vi "SecToCost.vi"(10 "Rate":dbl, 11 "Seconds":dbl) -> (3 "StoCcluster":T1)   [LabVIEW 2024]
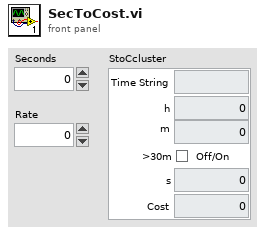
[diagram p1: front panel]
types:
  T1 = cluster{"Time String":string, "h":i32, "m":i32, ">30m":bool, "s":i32, "Cost":dbl}
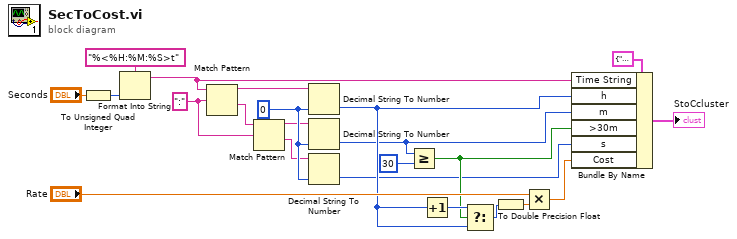
[diagram p0: block diagram]
diagram:
  w13 = ":" ("regular expression")
  w17 = 0 ("default (0 I32)")
  n1 = To Unsigned Quad Integer(1:"Seconds") -> (0:w10:u64)
  n2 = Format Into String(format string="%<%H:%M:%S>t", w10) -> (resulting string=w7:string)  [unwired: 2 in, 1 out]
  n3 = Match Pattern(string=w7, regular expression=w13) -> (before substring=w16:string, after substring=w18:string)  [unwired: 1 in, 2 out]
  n4 = Match Pattern(string=w18, regular expression=w13) -> (before substring=w14:string, after substring=w15:string)  [unwired: 1 in, 2 out]
  n5 = Decimal String To Number(string=w16, default (0L)=w17) -> (number=w6:i32)  [unwired: 1 in, 1 out]
  n6 = Decimal String To Number(string=w14, default (0L)=w17) -> (number=w5:i32)  [unwired: 1 in, 1 out]
  n7 = Decimal String To Number(string=w15, default (0L)=w17) -> (number=w1:i32)  [unwired: 1 in, 1 out]
  n8 = Greater Or Equal?(x=w5, y=30) -> (x >= y?=w4:bool)
  n9 = Increment(x=w6) -> (x+1=w22:i32)
  n10 = Select(t=w22, s=w4, f=w6) -> (s? t:f=w21:i32)
  n11 = To Double Precision Float(number=w21) -> (double precision float=w9:dbl)
  n12 = Multiply(x="Rate", y=w9) -> (x*y=w3:dbl)
  n13 = Bundle By Name(cluster=T1 {"Time String"="", "h"=0, "m"=0, ">30m"=FALSE, "s"=0, "Cost"=0.0} ("StoCcluster"), "Time String"=w7, "h"=w6, "m"=w5, ">30m"=w4, "s"=w1, "Cost"=w3) -> (→"StoCcluster":T1)
